vi "exec.vi"(8 "error in (no error)":errorcluster, 10 "context":refnum<class "IContextThisComponent.lvclass">, 11 "Command in":refnum<class "OnIncomingMessagingError.lvclass">) -> (0 "error out":errorcluster, 2 "context 2":refnum<class "IContextThisComponent.lvclass">, 3 "Command out":refnum<class "OnIncomingMessagingError.lvclass">)   [LabVIEW 2012, in "Commands.lvlib" / "OnIncomingMessagingError.lvclass"]
uses:
  OnIncomingMessagingError.lvclass
  IContextThisComponent/IContextThisComponent.lvclass
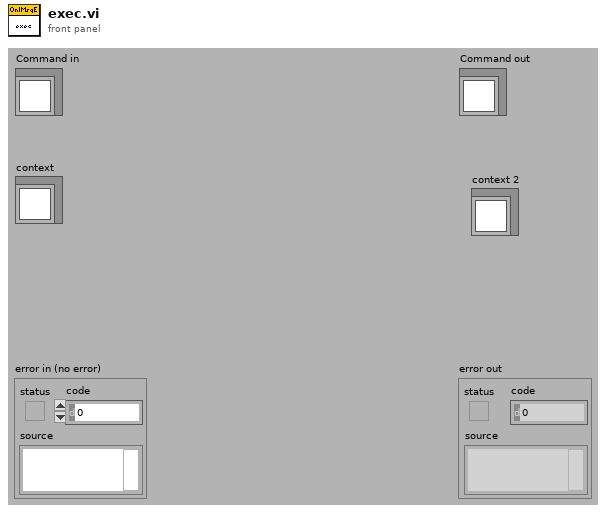
[diagram p1: front panel]
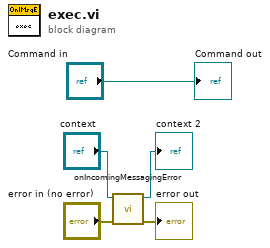
[diagram p0: block diagram]
diagram:
  n1 = call-dynamic "onIncomingMessagingError.vi"("error in (no error)"="error in (no error)", "IContextThisComponent in"="context") -> ("error out"=→"error out":errorcluster, "IContextThisComponent out"=→"context 2":refnum<class "IContextThisComponent.lvclass">)  [unwired: 8 in]
  "Command out" <- "Command in"
